vi "Pop up.vi"(8 "error in (no error)":errorcluster, 11 "Message In":string) -> (0 "error out":errorcluster)   [LabVIEW 2016, in "User Interface.lvlib"]
uses:
  User Interface.lvlib
panel:
  in  "OK":bool
  out "Message":string
  out "ATE Title":string
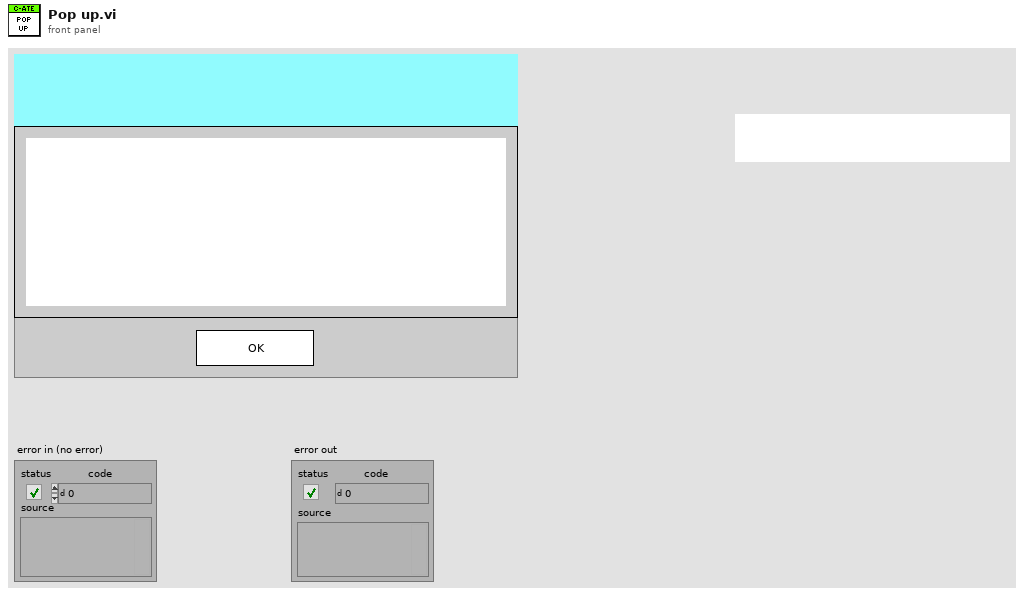
[diagram p1: front panel]
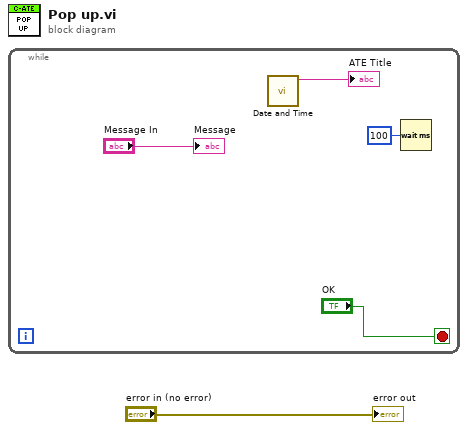
[diagram p0: block diagram]
diagram:
  n1 = while {
    stop <- "OK" stop-if-true
    n2 = call "Date and Time.vi"() -> ("Current Time"=→"ATE Title":string)  [unwired: 11 in]
    n3 = Wait (ms)(milliseconds to wait=u32 100) -> ()  [unwired: 1 out]
    "Message" <- "Message In"
  }
  "error out" <- "error in (no error)"
